vi "Wolna_przetwarzanie.vi"(6 "Rej Param":cluster{"Kanały":i32[][], T1[]}, 7 "Okres In":dbl, 8 "error in (no error)":errorcluster, 9 "Przetworzone in":T2, 11 "Wydzielone in":T2) -> (0 "error out":errorcluster, 1 "Przetworzone out":T2)   [LabVIEW 2013]
doc: "Use this template to build a VI to use as a subVI."
uses:
  Kontrolki/Przetwarzanie/Kanaly.ctl
  Kontrolki/GUI/RejWol_typ.ctl
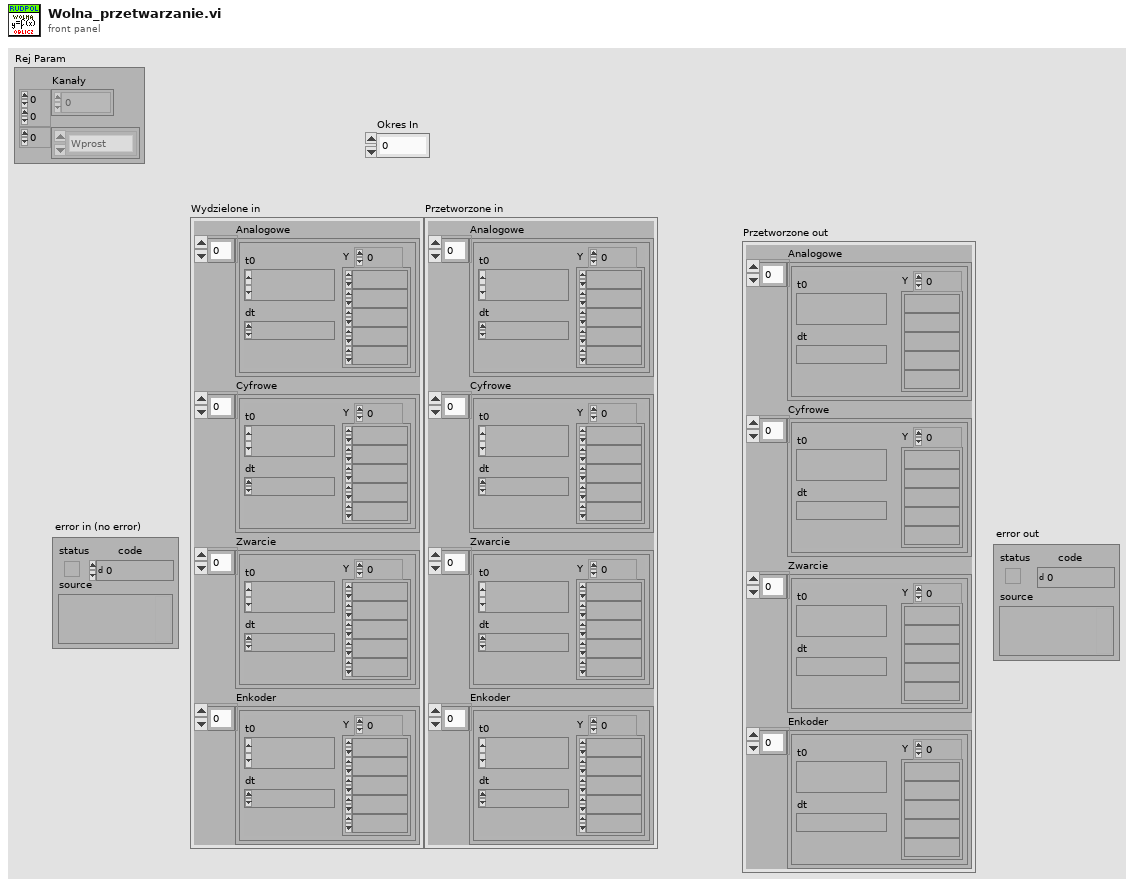
[diagram p1: front panel]
types:
  T1 = typedef "RejWol_typ.ctl" = enum16{"Wprost", "Moduł", "Kwadrat", "Iloczyn", "Faza"}
  T2 = typedef "Kanaly.ctl" = cluster{"Analogowe":waveform(dbl)[], "Cyfrowe":waveform(dbl)[], "Zwarcie":waveform(dbl)[], "Enkoder":waveform(dbl)[]}
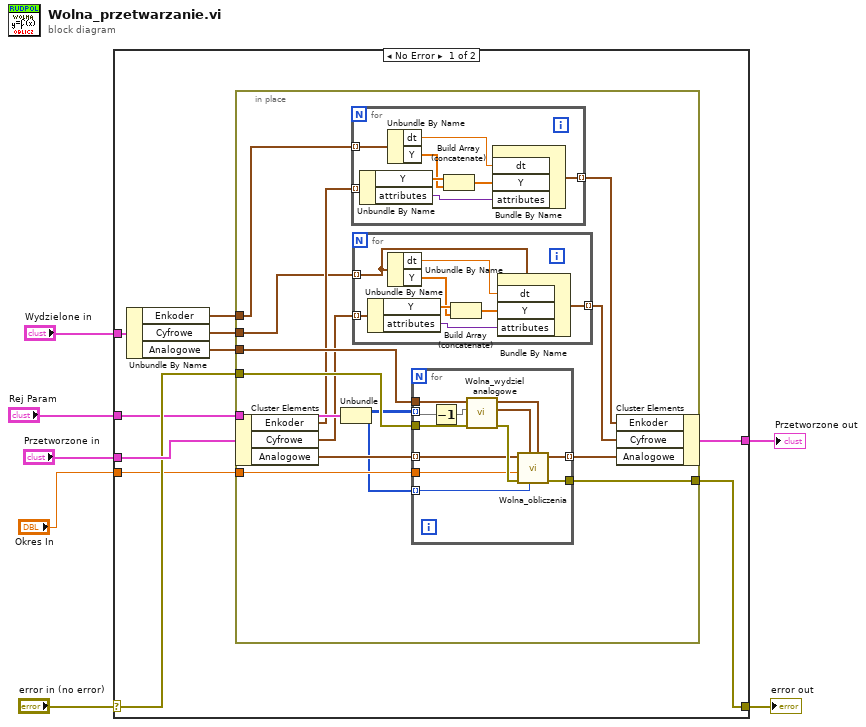
[diagram p0: block diagram]
diagram:
  n1 = case shown="No Error" "error in (no error)" {
    selector: "error in (no error)" -> [w13 w62]
    tunnel: [w12 w62] -> w6
    tunnel: "Wydzielone in" -> [w15 _]
    tunnel: "Przetworzone in" -> [w17 w61]
    tunnel: [w16 w61] -> w3
    tunnel: "Rej Param" -> [w11 _]
    tunnel: "Okres In" -> [w10 _]
    frame No Error {
      n2 = Unbundle By Name(w15) -> ("Enkoder"=w9:waveform(dbl)[], "Cyfrowe"=w8:waveform(dbl)[], "Analogowe"=w14:waveform(dbl)[])
      n3 = in-place {
        in-place-border: w14 -> [w28]
        in-place-border: w13 -> [w30]
        in-place-border: [w29] -> w12
        in-place-border: w11 -> [w26]
        in-place-border: w10 -> [w27]
        in-place-border: w9 -> [w23]
        in-place-border: w8 -> [w19]
        n4 = in-place-cluster #1(w17) -> ("Enkoder"=w22:waveform(dbl)[], "Cyfrowe"=w18:waveform(dbl)[], "Analogowe"=w32:waveform(dbl)[])
        n5 = Unbundle(w26) -> ("Kanały"=w25:i32[][], w24:T1[])
        n6 = for {
          tunnel: w23 -> [w42] mode=indexing
          tunnel: w22 -> [w43] mode=indexing
          tunnel: [w44] -> w21 mode=indexing
          n7 = Unbundle By Name(w43) -> ("Y"=w48:dbl[], "attributes"=w41:variant)
          n8 = Unbundle By Name(w42) -> ("dt"=w45:dbl, "Y"=w47:dbl[])
          n9 = Build Array (concatenate)(w48, w47) -> (w46:dbl[])
          n10 = Bundle By Name("dt"=w45, "Y"=w46, "attributes"=w41) -> (w44:waveform(dbl))  [unwired: 1 in]
        }
        n11 = for {
          tunnel: w19 -> [w34] mode=indexing
          tunnel: w18 -> [w35] mode=indexing
          tunnel: [w36] -> w20 mode=indexing
          n12 = Unbundle By Name(w35) -> ("Y"=w40:dbl[], "attributes"=w33:variant)
          n13 = Unbundle By Name(w34) -> ("dt"=w37:dbl, "Y"=w39:dbl[])
          n14 = Build Array (concatenate)(w40, w39) -> (w38:dbl[])
          n15 = Bundle By Name(cluster=w34, "dt"=w37, "Y"=w38, "attributes"=w33) -> (w36:waveform(dbl))
        }
        n16 = for {
          tunnel: w32 -> [w57] mode=indexing
          tunnel: [w56] -> w31 mode=indexing
          tunnel: w30 -> [w55]
          tunnel: [w54] -> w29
          tunnel: w28 -> [w53]
          tunnel: w25 -> [w50] mode=indexing
          tunnel: w27 -> [w52]
          tunnel: w24 -> [w51] mode=indexing
          n17 = Decrement(x=w50) -> (x-1=w49:i32[])
          n18 = call "Wolna_wydziel analogowe.vi"("error in (no error)"=w55, "Kanaly in"=w49, "Analogowe in"=w53) -> ("error out"=w60:errorcluster, "wybrany 2"=w58:waveform(dbl), "wybrany 1"=w59:waveform(dbl))  [unwired: 6 in]
          n19 = call "Wolna_obliczenia.vi"("Wektor1 in"=w59, "Typ rejestracji"=w51, "Wektor2 in"=w58, "error in (no error)"=w60, "Okres"=w52, "Wolna in"=w57) -> ("error out"=w54:errorcluster, "Wolna out"=w56:waveform(dbl))  [unwired: 3 in, 1 out]
        }
        n20 = in-place-cluster #1("Enkoder"=w21, "Cyfrowe"=w20, "Analogowe"=w31) -> (w16:T2)
      }
    }
    frame Error {
    }
  }
  "error out" <- w6
  "Przetworzone out" <- w3
